vi "Cleanup.vi"(8 "error in (no error)":errorcluster, 11 "UIMessage in":refnum<class "UIMessage.lvclass">) -> (0 "error out":errorcluster)   [LabVIEW 2020, in "TSnax.lvlib" / "UIMessage.lvclass"]
uses:
  UIMessage.lvclass
  UIMessage.lvclass/UIMessage.ctl
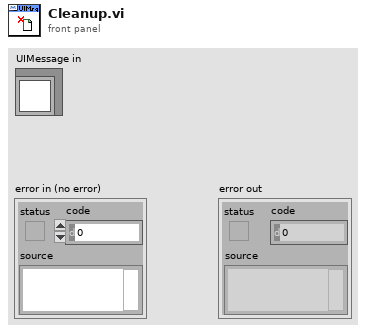
[diagram p1: front panel]
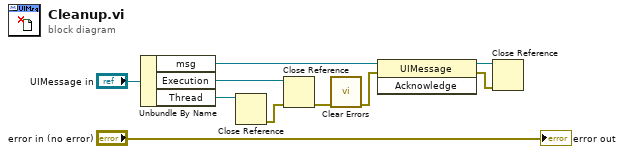
[diagram p0: block diagram]
diagram:
  n1 = Unbundle By Name("UIMessage in") -> ("msg"=w3:refnum<k7>, "Execution"=w2:refnum<k7>, "Thread"=w1:refnum<k7>)
  n2 = Close Reference(reference=w1) -> (error out=w9:errorcluster)  [unwired: 1 in]
  n3 = Close Reference(reference=w2, error in (no error)=w9) -> (error out=w8:errorcluster)
  n4 = call <vilib>:"Clear Errors.vi"("error in (no error)"=w8) -> ("error out"=w7:errorcluster)  [unwired: 5 in, 1 out]
  n5 = invoke class="UIMessage" method="Acknowledge"(reference=w3, error in=w7) -> (reference out=w5:refnum<k7>, error out=w6:errorcluster)  [unwired: 1 in, 1 out]
  n6 = Close Reference(reference=w5, error in (no error)=w6) -> ()  [unwired: 1 out]
  "error out" <- "error in (no error)"
